vi "pr1a1.vi"() -> ()   [LabVIEW 2013]
uses:
  <vilib>/Utility/error.llb/DialogType.ctl
  <vilib>/DAQmx/write.llb/DAQmx Write (Analog 1D DBL 1Chan NSamp).vi
  <vilib>/DAQmx/create/channels.llb/DAQmx Create Channel (AO-Voltage-Basic).vi
  <vilib>/DAQmx/configure/timing.llb/DAQmx Timing (Sample Clock).vi
  <vilib>/Utility/file.llb/Read From Spreadsheet File (DBL).vi
  <vilib>/DAQmx/miscellaneous.llb/DAQmx Fill In Error Info.vi
panel:
  in  "Canal generar":tag
  in  "Valor maximo generar":dbl=10.0 format="%0.2f"
  in  "Valor minimo generar":dbl=-10.0 format="%0.2f"
  in  "rate m/s generar":dbl=1000.0 format="%0.2f"
  out "grafico de datos generados 2":waveform(dbl)(graph)
  out "Grafico de datos generados":waveform(dbl)(graph)
  in  "muestras por canal generar":i32=1000
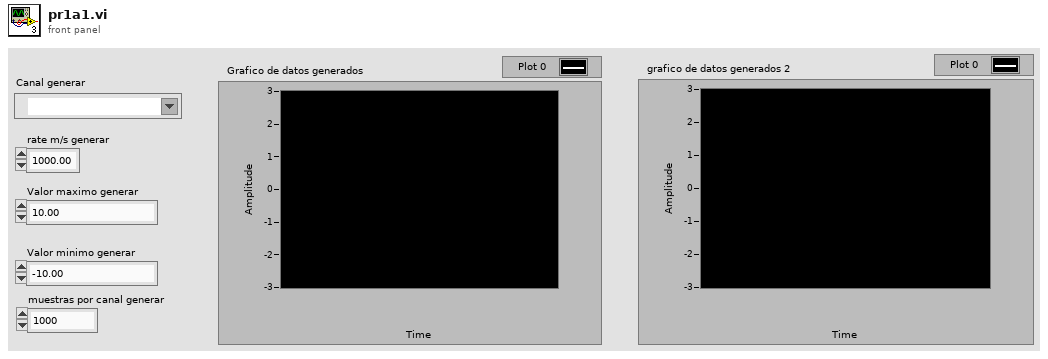
[diagram p1: front panel]
types:
  T1 = typedef "DialogType.ctl" = u16
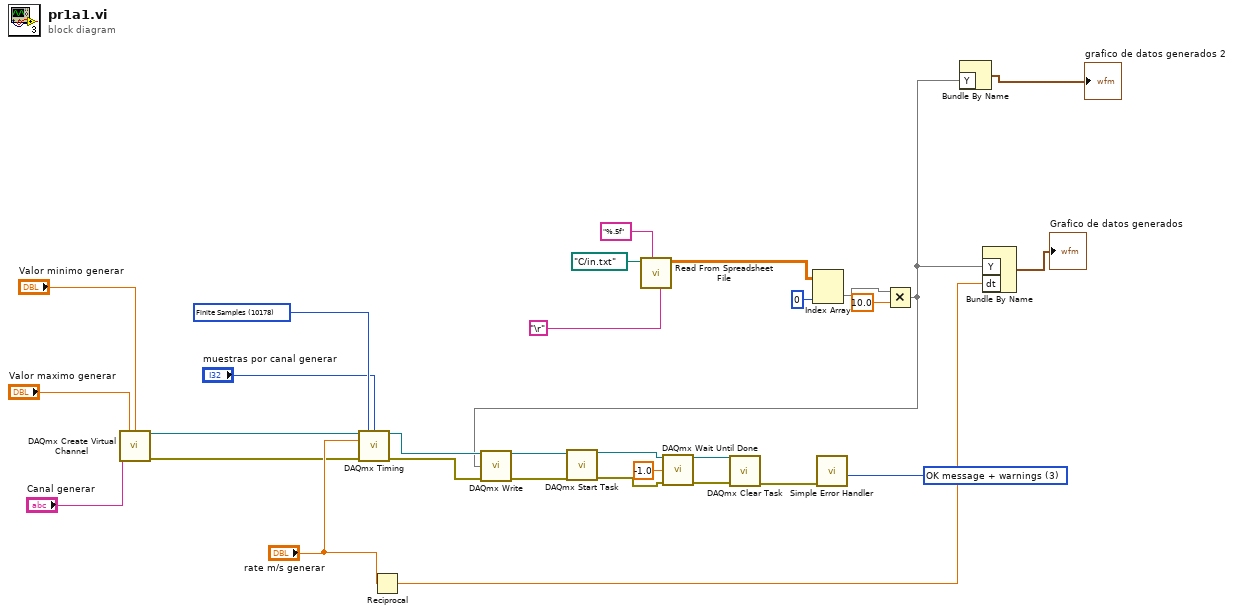
[diagram p0: block diagram]
diagram:
  w3 = T1 3 items=["no dialog", "OK message", "continue or stop message", "OK message + warnings", "continue/stop + warnings"] ("type of dialog (OK msg:1)")
  w20 = 10178 items=["Finite Samples"=10178, "Continuous Samples"=10123, "Hardware Timed Single Point"=12522] ("sample mode")
  n1 = call-poly <vilib>:"DAQmx Create Virtual Channel.vi"("maximum value"="Valor maximo generar", "minimum value"="Valor minimo generar", "physical channels"="Canal generar") -> ("task out"=w5:refnum<k21>, "error out"=w4:errorcluster)  [unwired: 11 in]
  n2 = call-poly <vilib>:"DAQmx Timing.vi"("task/channels in"=w5, "sample mode"=w20, "samples per channel"="muestras por canal generar", "rate"="rate m/s generar", "error in"=w4) -> ("task out"=w24:refnum<k21>, "error out"=w17:errorcluster)  [unwired: 9 in]
  n3 = Reciprocal(x="rate m/s generar") -> (1/x=w10:dbl)
  n4 = call-poly <vilib>:"Read From Spreadsheet File.vi"("delimiter (\\t)"="\r", "format (%.3f)"="%.5f", "file path (dialog if empty)"=path "C:/in.txt") -> ("all rows"=w18:dbl[][])  [unwired: 4 in, 4 out]
  n5 = Index Array(array=w18, index (col)=0 ("disabled index (col)")) -> (element=w26:dbl[])  [unwired: 1 in]
  n6 = Multiply(x=w26, y=10.0) -> (x*y=w11:dbl[])
  n7 = call-poly <vilib>:"DAQmx Write.vi"("task/channels in"=w24, "data"=w11, "error in"=w17) -> ("task out"=w23:refnum<k21>, "error out"=w16:errorcluster)  [unwired: 10 in, 1 out]
  n8 = call <vilib>:"DAQmx Start Task.vi"("task/channels in"=w23, "error in"=w16) -> ("task out"=w22:refnum<k21>, "error out"=w15:errorcluster)  [unwired: 12 in]
  n9 = call <vilib>:"DAQmx Wait Until Done.vi"("task/channels in"=w22, "timeout (sec)"=-1.0, "error in"=w15) -> ("task out"=w21:refnum<k21>, "error out"=w14:errorcluster)  [unwired: 11 in]
  n10 = call <vilib>:"DAQmx Clear Task.vi"("task in"=w21, "error in"=w14) -> ("error out"=w9:errorcluster)  [unwired: 13 in]
  n11 = call <vilib>:"Simple Error Handler.vi"("type of dialog (OK msg:1)"=w3, "error in (no error)"=w9) -> ()  [unwired: 3 in, 5 out]
  n12 = Bundle By Name("Y"=w11) -> (→"grafico de datos generados 2":waveform(dbl))  [unwired: 1 in]
  n13 = Bundle By Name("Y"=w11, "dt"=w10) -> (→"Grafico de datos generados":waveform(dbl))  [unwired: 1 in]
